vi "Global_ACT_Data Out.vi"() -> ()   [LabVIEW 2020, in "Shooter_ACT.lvlib"]
uses:
  roboRIO Code/Systems/Shooter/Shooter_ACT.lvlib
  roboRIO Code/Systems/Shooter/Cluster_Shooter Status.ctl
  roboRIO Code/Systems/Shooter/Cluster_Speed Sensor Values.ctl
  roboRIO Code/Systems/Shooter/Cluster_Velocity Values.ctl
  roboRIO Code/Systems/Shooter/Cluster_Voltage Values.ctl
  <vilib>/Rock Robotics/WPI/ThirdParty/Phoenix-LabVIEW/Motor Controller/Controls/CTRE_Phoenix_MotorControl_ControlMode.ctl
panel:
  in  "ACT_Shooter_Control Mode":T1 items=["PercentOutput"=0, "Position"=1, "Velocity"=2, "Current"=3, "Follower"=5, "MotionProfile"=6, "MotionMagic"=7, "MotionProfileArc"=10, "Disabled"=15]
  in  "ACT_Shooter_Status":T2
  in  "ACT_Shooter Motor Value":dbl
  in  "ACT_Shooter_CycleTime(S)":dbl
  # "The Names of the Data items in the Global Variable MUST describe who the Single Writer is\nFor Actuator Globals the the naming convention is\n   \nACT_Lib Name_Data Name\n\nExamples:\nACT_Drive_X axis\nACT_Hopper_AgitatorSpeed"
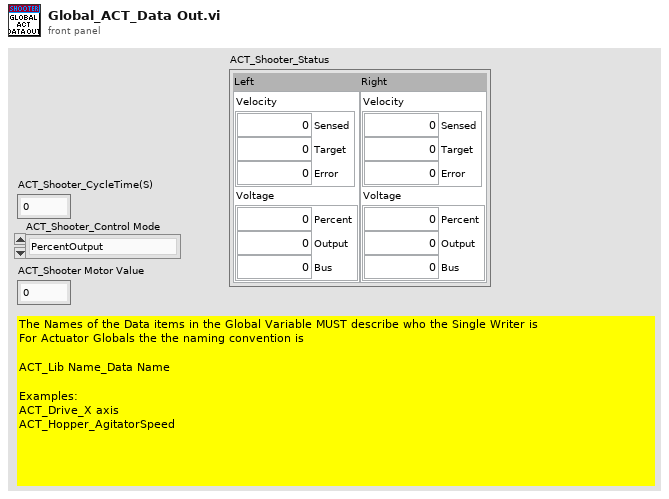
[diagram p1: front panel]
types:
  T1 = typedef "CTRE_Phoenix_MotorControl_ControlMode.ctl" = u16
  T2 = typedef "Shooter_ACT.lvlib/Cluster_Shooter Status.ctl" = cluster{"Left":T3, "Right":T3}
  T3 = typedef "Cluster_Speed Sensor Values.ctl" = cluster{"Velocity":T4, "Voltage":T5}
  T4 = typedef "Shooter_ACT.lvlib/Cluster_Velocity Values.ctl" = cluster{"Sensed":dbl, "Target":dbl, "Error":dbl}
  T5 = typedef "Shooter_ACT.lvlib/Cluster_Voltage Values.ctl" = cluster{"Percent":dbl, "Output":dbl, "Bus":dbl}
diagram:
